vi "Drive Controller.vi"(8 "error in":errorcluster) -> ()   [LabVIEW 2020]
doc: "This VI executes continuously carrying out the current operation and responding to updates or new operation requests. It will often contain the timing or control code that is difficult to place directly in TeleOp. This VI generally opens all sensors and motors and isolates the rest of the robot code from knowing implementation details of how the operations are carried out."
uses:
  <vilib>/Rock Robotics/WPI/Framework/Completion Status.ctl
  Drive Setpoints.ctl
  Drive Operations.ctl
  <vilib>/Rock Robotics/WPI/SafetyOutput/WPI_SafetyOutputConfigMenu.ctl
  <vilib>/Rock Robotics/WPI/RobotDrive/WPI_RobotDriveOpen2MotorWithExistingMotors.vi
  <vilib>/Rock Robotics/Network Tables/NT Write Numeric Array.vi
  <vilib>/Rock Robotics/WPI/ThirdParty/REV Robotics/REVLib/Typedef/Spark MAX Motor Type.ctl
  <vilib>/Rock Robotics/WPI/ThirdParty/REV Robotics/REVLib/Typedef/Spark MAX Idle Mode.ctl
panel:
  in  "Interactive Values":T1
  in  "Buttons":cluster{"Execute Cmd":bool, "Abort Cmd":bool}
  out "Command Timing":cluster{"Start Time (ms)":u32, "Iterations":i32}
  out "Status":T3
  out "Setpoints":T4(graph)
  out "Current\nCmd":string
  # "Tip: The graph shows the motor setpoints. It may also be helpful to observe inputs and sensor values.\nYou may also want to display tuning or debugging controls."
  # "Interactive Command: You may fill in the settings for a command\nand schedule it with the Execute button. You can observe and abort\nany command while fine tuning the code for the controller."
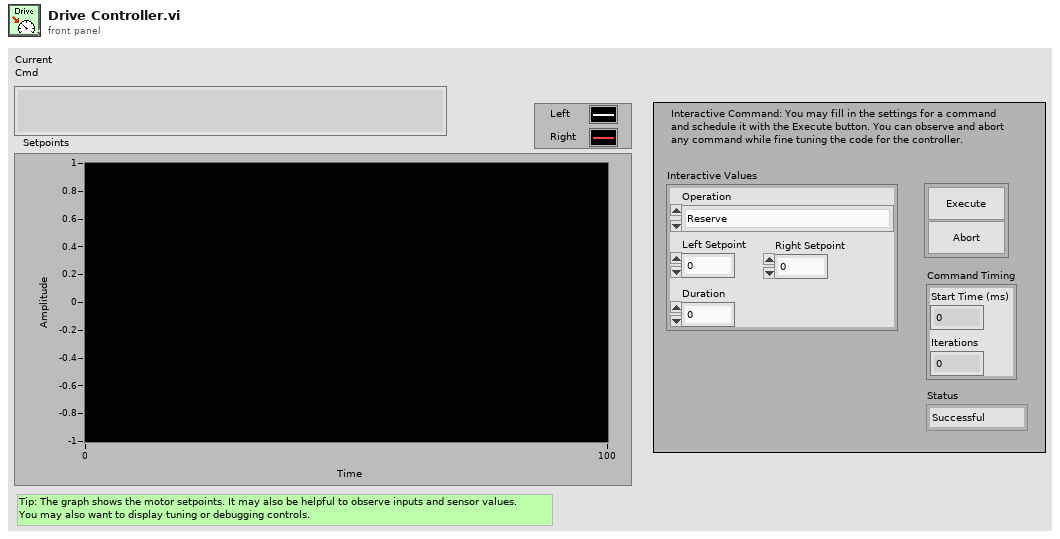
[diagram p1: front panel]
types:
  T1 = typedef "Drive Setpoints.ctl" = cluster{"Operation":T2, "Left Setpoint":dbl, "Right Setpoint":dbl, "Duration":dbl}
  T2 = typedef "Drive Operations.ctl" = enum16{"Reserve", "Read Current", "Immediate", "Drive for Time", "Drive for Distance"}
  T3 = typedef "Completion Status.ctl" = enum16{"Successful", "Aborted", "Incomplete"}
  T4 = cluster{"Left Setpoint":dbl, "Right Setpoint":dbl}
  T5 = typedef "WPI_SafetyOutputConfigMenu.ctl" = enum16{"Enable", "Disable"}
  T6 = typedef "WPI_MotorControlDeviceRef.ctl" = cluster{"DeviceStatus":errorcluster, "Type":T7, "PWM":cluster{"PWM Channel":T8, "DeadBand":T9}, "CAN":cluster{"Device Number":u8, "SetOutput VI Ref":variant, "GetOutput VI Ref":variant, "Enable VI Ref":variant, "Disable VI Ref":variant, "Data":variant}, "Invert":bool, "DIO PWM":cluster{"PWM \"Enable\" Channel":T8, "DIOChannel":T10, "PWM Rate":dbl}}
  T7 = typedef "WPI_MotorControlType.ctl" = enum16{"PWM", "CAN", "DIO PWM"}
  T8 = typedef "FPGA_DIOPWMChannel.ctl" = enum8{"PWM 0", "PWM 1", "PWM 2", "PWM 3", "PWM 4", "PWM 5", "PWM 6", "PWM 7", "PWM 8", "PWM 9", "PWM MXP 0", "PWM MXP 1", "PWM MXP 2", "PWM MXP 3", "PWM MXP 4", "PWM MXP 5", "PWM MXP 6", "PWM MXP 7", "PWM MXP 8", "PWM MXP 9", "Invalid"}
  T9 = typedef "WPI_PWMDeadband.ctl" = cluster{"Name":string, "maxPositivePwm":i32, "minPositivePwm":i32, "centerPwm":i32, "maxNegativePwm":i32, "minNegativePwm":i32, "angularRange":u16}
  T10 = typedef "FPGA_DIOChannel.ctl" = enum8{"DIO 0", "DIO 1", "DIO 2", "DIO 3", "DIO 4", "DIO 5", "DIO 6", "DIO 7", "DIO 8", "DIO 9", "DIO MXP 0", "DIO MXP 1", "DIO MXP 2", "DIO MXP 3", "DIO MXP 4", "DIO MXP 5", "DIO MXP 6", "DIO MXP 7", "DIO MXP 8", "DIO MXP 9", "DIO MXP 10", "DIO MXP 11", "DIO MXP 12", "DIO MXP 13", "DIO MXP 14", "DIO MXP 15", "SPI Port CS1", "SPI Port CS2", "SPI Port CS3", "SPI Port MISO", "SPI Port MOSI", "Invalid"}
  T11 = typedef "Spark MAX Idle Mode.ctl" = enum16{"Coast", "Brake"}
  T12 = typedef "Spark MAX Motor Type.ctl" = enum16{"Brushed", "Brushless"}
  T13 = typedef "WPI_RobotDriveDevRef.ctl" = cluster{"DevStatus":errorcluster, "Motors[]":T6[], "Square Inputs":bool, "Max Output":dbl}
  T14 = typedef "Command Status Info.ctl" = cluster{"Name":string, "Status":T3, "notifier out":T15}
  T15 = typedef "Completion Notifier.ctl" = refnum<notifier>
  T16 = cluster{"SubSystem Data":T1, cluster{"Start Time (ms)":u32, "Iterations":i32}, cluster{"Command Info":T14, "Description":string, "Default Command":T1, "queue out":refnum<queue>, "Subsystem Name":string}}
  T17 = cluster{"SubSystem Data":T1, cluster{"Start Time (ms)":u32, "Iterations":i32}, "Default Command Arguments":cluster{"Command Info":T14, "Description":string, "Default Command":T1, "queue out":refnum<queue>, "Subsystem Name":string}}
  T18 = cluster{"Don't move motors while reserved":dbl, "Don't move motors while reserved":dbl}
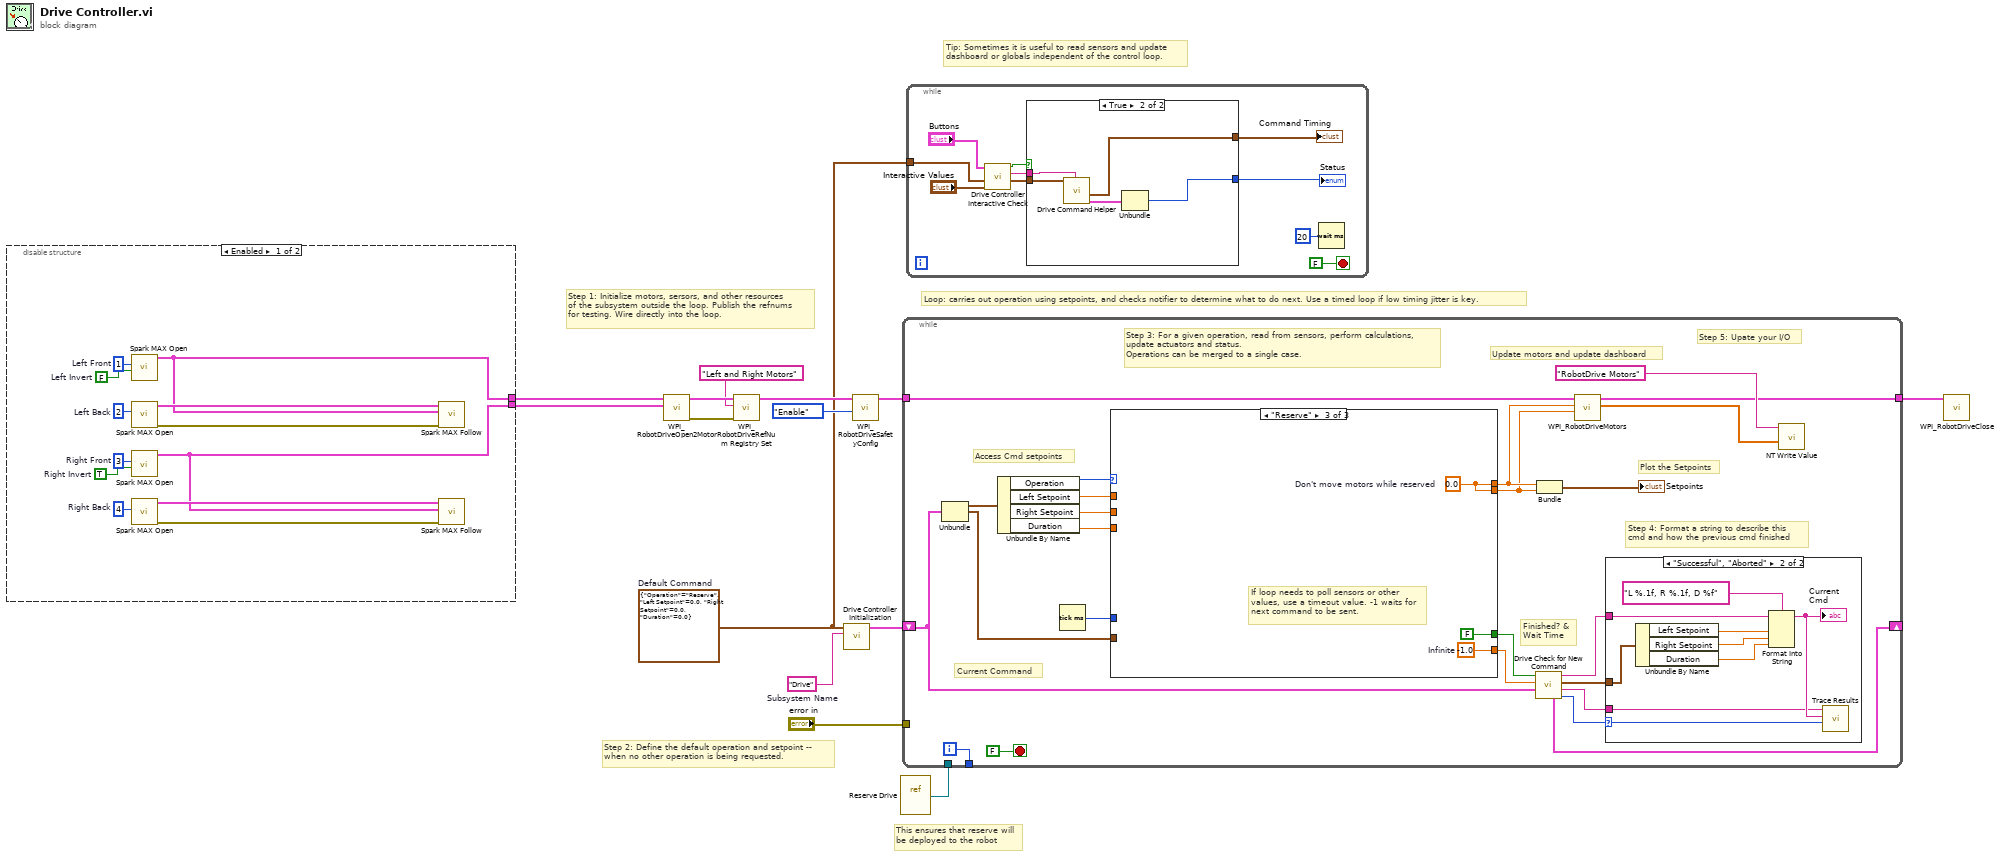
[diagram p0: block diagram]
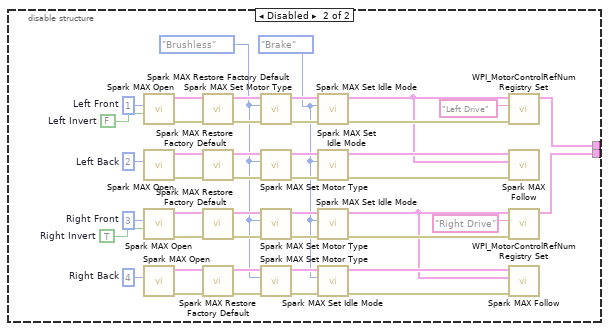
[diagram p2: hidden frame]
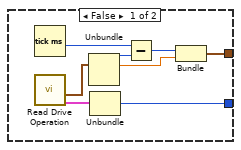
[diagram p3: hidden frame]
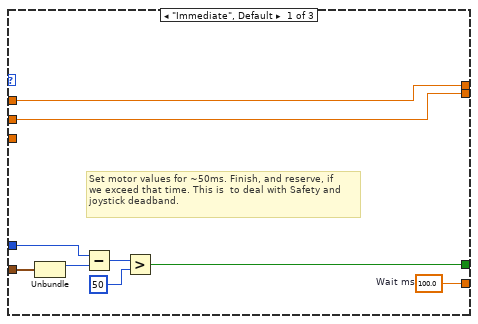
[diagram p5: hidden frame]
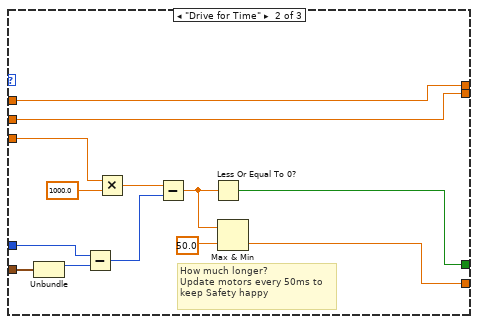
[diagram p6: hidden frame]
diagram:
  w4 = T1 {"Operation"=enum."Reserve", "Left Setpoint"=0.0, "Right Setpoint"=0.0, "Duration"=0.0}  # Default Command
  w14 = "Drive"  # Subsystem Name
  # "This ensures that reserve will\nbe deployed to the robot"
  # "Tip: Sometimes it is useful to read sensors and update\ndashboard or globals independent of the control loop."
  # "Step 2: Define the default operation and setpoint --\nwhen no other operation is being requested."
  # "Step 1: Initialize motors, sersors, and other resources\nof the subsystem outside the loop. Publish the refnums\nfor testing. Wire directly into the loop."
  # "Loop: carries out operation using setpoints, and checks notifier to determine what to do next. Use a timed loop if low timing jitter is key."
  n1 = disable-structure shown="Enabled" {
    disable-tunnel: [w15 w30] -> w3
    disable-tunnel: [w17 w29] -> w2
    frame Enabled {
      w19 = u8 4  # Right Back
      w20 = u8 3  # Right Front
      w21 = u8 2  # Left Back
      w22 = u8 1  # Left Front
      w23 = TRUE  # Right Invert
      w24 = FALSE  # Left Invert
      n2 = call <vilib>:"Spark MAX Open.vi"("Invert"=w24, "Device Number"=w22) -> ("MotorControlDeviceRef"=w15:T6)  [unwired: 8 in, 1 out]
      n3 = call <vilib>:"Spark MAX Open.vi"("Device Number"=w21) -> ("error out"=w26:errorcluster, "MotorControlDeviceRef"=w16:T6)  [unwired: 9 in]
      n4 = call <vilib>:"Spark MAX Open.vi"("Invert"=w23, "Device Number"=w20) -> ("MotorControlDeviceRef"=w17:T6)  [unwired: 8 in, 1 out]
      n5 = call <vilib>:"Spark MAX Open.vi"("Device Number"=w19) -> ("error out"=w25:errorcluster, "MotorControlDeviceRef"=w18:T6)  [unwired: 9 in]
      n6 = call <vilib>:"Spark MAX Follow.vi"("error in (no error)"=w26, "Master Controller"=w15, "MotorControlDeviceRef"=w16) -> ()  [unwired: 7 in, 2 out]
      n7 = call <vilib>:"Spark MAX Follow.vi"("error in (no error)"=w25, "Master Controller"=w17, "MotorControlDeviceRef"=w18) -> ()  [unwired: 7 in, 2 out]
    }
    frame Disabled {
      w27 = Spark_MAX_Idle_Mode."Brake" ("Idle Mode")
      w28 = Spark_MAX_Motor_Type."Brushless" ("Motor Type")
      w37 = u8 4  # Right Back
      w38 = u8 3  # Right Front
      w39 = u8 2  # Left Back
      w40 = u8 1  # Left Front
      w41 = TRUE  # Right Invert
      w42 = FALSE  # Left Invert
      n8 = call <vilib>:"Spark MAX Open.vi"("Invert"=w42, "Device Number"=w40) -> ("error out"=w70:errorcluster, "MotorControlDeviceRef"=w69:T6)  [unwired: 8 in]
      n9 = call <vilib>:"Spark MAX Open.vi"("Device Number"=w39) -> ("error out"=w59:errorcluster, "MotorControlDeviceRef"=w60:T6)  [unwired: 9 in]
      n10 = call <vilib>:"Spark MAX Open.vi"("Invert"=w41, "Device Number"=w38) -> ("error out"=w53:errorcluster, "MotorControlDeviceRef"=w54:T6)  [unwired: 8 in]
      n11 = call <vilib>:"Spark MAX Open.vi"("Device Number"=w37) -> ("error out"=w48:errorcluster, "MotorControlDeviceRef"=w47:T6)  [unwired: 9 in]
      n12 = call <vilib>:"Spark MAX Restore Factory Default.vi"("error in"=w70, "MotorControlDeviceRef"=w69) -> ("error out"=w68:errorcluster, "MotorControlDeviceRef"=w67:T6)  [unwired: 8 in]
      n13 = call <vilib>:"Spark MAX Restore Factory Default.vi"("error in"=w59, "MotorControlDeviceRef"=w60) -> ("error out"=w61:errorcluster, "MotorControlDeviceRef"=w62:T6)  [unwired: 8 in]
      n14 = call <vilib>:"Spark MAX Restore Factory Default.vi"("error in"=w53, "MotorControlDeviceRef"=w54) -> ("error out"=w55:errorcluster, "MotorControlDeviceRef"=w56:T6)  [unwired: 8 in]
      n15 = call <vilib>:"Spark MAX Restore Factory Default.vi"("error in"=w48, "MotorControlDeviceRef"=w47) -> ("error out"=w46:errorcluster, "MotorControlDeviceRef"=w45:T6)  [unwired: 8 in]
      n16 = call <vilib>:"Spark MAX Set Motor Type.vi"("error in (no error)"=w68, "Motor Type"=w28, "MotorControlDevRef"=w67) -> ("error out"=w66:errorcluster, "MotorControlDeviceRef"=w65:T6)  [unwired: 7 in]
      n17 = call <vilib>:"Spark MAX Set Motor Type.vi"("error in (no error)"=w61, "Motor Type"=w28, "MotorControlDevRef"=w62) -> ("error out"=w63:errorcluster, "MotorControlDeviceRef"=w64:T6)  [unwired: 7 in]
      n18 = call <vilib>:"Spark MAX Set Motor Type.vi"("error in (no error)"=w55, "Motor Type"=w28, "MotorControlDevRef"=w56) -> ("error out"=w57:errorcluster, "MotorControlDeviceRef"=w58:T6)  [unwired: 7 in]
      n19 = call <vilib>:"Spark MAX Set Motor Type.vi"("error in (no error)"=w46, "Motor Type"=w28, "MotorControlDevRef"=w45) -> ("error out"=w44:errorcluster, "MotorControlDeviceRef"=w43:T6)  [unwired: 7 in]
      n20 = call <vilib>:"Spark MAX Set Idle Mode.vi"("error in (no error)"=w66, "Idle Mode"=w27, "MotorControlDeviceRef in"=w65) -> ("error out"=w36:errorcluster, "MotorControlDeviceRef out"=w34:T6)  [unwired: 7 in]
      n21 = call <vilib>:"Spark MAX Set Idle Mode.vi"("error in (no error)"=w63, "Idle Mode"=w27, "MotorControlDeviceRef in"=w64) -> ("error out"=w52:errorcluster, "MotorControlDeviceRef out"=w51:T6)  [unwired: 7 in]
      n22 = call <vilib>:"Spark MAX Set Idle Mode.vi"("error in (no error)"=w57, "Idle Mode"=w27, "MotorControlDeviceRef in"=w58) -> ("error out"=w35:errorcluster, "MotorControlDeviceRef out"=w33:T6)  [unwired: 7 in]
      n23 = call <vilib>:"Spark MAX Set Idle Mode.vi"("error in (no error)"=w44, "Idle Mode"=w27, "MotorControlDeviceRef in"=w43) -> ("error out"=w49:errorcluster, "MotorControlDeviceRef out"=w50:T6)  [unwired: 7 in]
      n24 = call <vilib>:"WPI_MotorControlRefNum Registry Set.vi"("error in (no error)"=w36, "refnum name"="Left Drive", "MotorControlDevRef"=w34) -> ("MotorControlDevRef"=w30:T6)  [unwired: 7 in, 1 out]
      n25 = call <vilib>:"Spark MAX Follow.vi"("error in (no error)"=w52, "Master Controller"=w34, "MotorControlDeviceRef"=w51) -> ()  [unwired: 7 in, 2 out]
      n26 = call <vilib>:"WPI_MotorControlRefNum Registry Set.vi"("error in (no error)"=w35, "refnum name"="Right Drive", "MotorControlDevRef"=w33) -> ("MotorControlDevRef"=w29:T6)  [unwired: 7 in, 1 out]
      n27 = call <vilib>:"Spark MAX Follow.vi"("error in (no error)"=w49, "Master Controller"=w33, "MotorControlDeviceRef"=w50) -> ()  [unwired: 7 in, 2 out]
    }
  }
  n28 = call-poly <vilib>:"WPI_RobotDriveOpen2Motor.vi"("Right Motor Dev Ref"=w2, "Left Motor Dev Ref"=w3) -> ("error out"=w11:errorcluster, "RobotDriveDevRef"=w13:T13)  [unwired: 3 in, 5 out]
  n29 = call <vilib>:"WPI_RobotDriveRefNum Registry Set.vi"("error in (no error)"=w11, "refnum name"="Left and Right Motors", "RobotDriveDevRef"=w13) -> ("RobotDriveDevRef"=w10:T13)  [unwired: 1 in, 7 out]
  n30 = call "Drive Controller Initialization.vi"("Subsystem Name"=w14, "Default Command"=w4) -> ("Current Command"=w6:T16)  [unwired: 9 in]
  n31 = call <vilib>:"WPI_RobotDriveSafetyConfig.vi"("mode"=WPI_SafetyOutputConfigMenu."Enable", "RobotDriveDevRef"=w10) -> ("RobotDriveDevRef"=w8:T13)  [unwired: 8 in, 1 out]
  n32 = vi-ref "Reserve Drive.vi"() -> (w5:refnum<vi>)
  n33 = while {
    shift-right: [w81] -> _
    shift-left: w6 -> [w74]
    tunnel: [w93] -> _
    tunnel: w8 -> [w89]
    tunnel: "error in" -> [_]
    tunnel: w5 -> [_]
    tunnel: [w71] -> w1
    i -> [w93]
    stop <- FALSE stop-if-true
    # "Step 5: Upate your I/O"
    # "Step 4: Format a string to describe this\ncmd and how the previous cmd finished"
    # "Current Command"
    # "Update motors and update dashboard"
    # "Plot the Setpoints"
    # "Access Cmd setpoints"
    # "Finished? &\nWait Time"
    # "Step 3: For a given operation, read from sensors, perform calculations,\nupdate actuators and status.\nOperations can be merged to a single case."
    n34 = Unbundle(w74) -> ("SubSystem Data"=w88:T1, w75:cluster{"Start Time (ms)":u32, "Iterations":i32})  [unwired: 1 out]
    n35 = Unbundle By Name(w88) -> ("Operation"=w87:T2, "Left Setpoint"=w86:dbl, "Right Setpoint"=w85:dbl, "Duration"=w84:dbl)
    n36 = Tick Count (ms)() -> (millisecond timer value=w83:u32)
    n37 = case shown="\"Reserve\"" w87 {
      tunnel: [w112 w113 w128] -> w80
      tunnel: [w105 w120 FALSE ("ignore previous (F)")] -> w79
      tunnel: w75 -> [w104 w122 _]
      tunnel: [w111 w119 w126] -> w91
      tunnel: [w110 w118 w126] -> w90
      tunnel: w86 -> [w111 w119 _]
      tunnel: w85 -> [w110 w118 _]
      tunnel: w84 -> [_ w117 _]
      tunnel: w83 -> [w106 w116 _]
      frame "Immediate", Default {
        w112 = 100.0  # Wait ms
        # "Set motor values for ~50ms. Finish, and reserve, if\nwe exceed that time. This is  to deal with Safety and\njoystick deadband."
        n38 = Unbundle(w104) -> ("Start Time (ms)"=w107:u32)  [unwired: 1 out]
        n39 = Subtract(x=w106, y=w107) -> (x-y=w108:u32)
        n40 = Greater?(x=w108, y=u8 50 ("Left Motor")) -> (0:w105:bool)
      }
      frame "Drive for Time" {
        # "How much longer?\nUpdate motors every 50ms to\nkeep Safety happy"
        n41 = Unbundle(w122) -> ("Start Time (ms)"=w121:u32)  [unwired: 1 out]
        n42 = Subtract(x=w116, y=w121) -> (x-y=w125:u32)
        n43 = Multiply(x=w117, y=1000.0) -> (x*y=w124:dbl)
        n44 = Subtract(x=w124, y=w125) -> (x-y=w115:dbl)
        n45 = Less Or Equal To 0?(x=w115) -> (x <= 0?=w120:bool)
        n46 = Max & Min(x=w115, y=50.0) -> (min(x,y)=w113:dbl)  [unwired: 1 out]
      }
      frame "Reserve" {
        w126 = 0.0  # Don't move motors while reserved
        w128 = -1.0  # Infinite
        # "If loop needs to poll sensors or other\nvalues, use a timeout value. -1 waits for\nnext command to be sent."
      }
    }
    n47 = call "Drive Check for New Command.vi"("input cluster"=w74, "Wait time (ms)"=w80, "Finished?"=w79) -> ("Completion"=w82:T3, "Subsystem Name"=w76:string, "Current Command"=w77:T1, "Initial Trace String"=w78:string, "Next Command"=w81:T17)  [unwired: 4 in]
    n48 = Bundle("Don't move motors while reserved"=w91, "Don't move motors while reserved"=w90) -> (→"Setpoints":T18)  [unwired: 1 in]
    n49 = call <vilib>:"WPI_RobotDriveMotors.vi"("RightSpeed"=w90, "LeftSpeed"=w91, "RobotDriveDevRef"=w89) -> ("Motor Values"=w72:dbl[], "RobotDriveDevRef"=w71:T13)  [unwired: 1 in, 6 out]
    n50 = case shown="\"Successful\", \"Aborted\"" w82 {
      selector: w82 -> [_ w103]
      tunnel: w78 -> [_ w98]
      tunnel: w77 -> [_ w99]
      tunnel: w76 -> [_ w95]
      frame "Incomplete", Default {
        # "Continuing current command"
      }
      frame "Successful", "Aborted" {
        # "Report and setup for next command"
        n51 = Unbundle By Name(w99) -> ("Left Setpoint"=w101:dbl, "Right Setpoint"=w102:dbl, "Duration"=w96:dbl)
        n52 = Format Into String(format string="L %.1f, R %.1f, D %f", initial string=w98, w101, w102, w96) -> (resulting string=w97:string)  [unwired: 1 in, 1 out]
        "Current\nCmd" <- w97
        n53 = call <vilib>:"Trace Results.vi"("Status of previous command"=w103, "Description"=w97, "Subsystem"=w95) -> ()  [unwired: 9 in]
      }
    }
    n54 = call-poly <vilib>:"NT Write Value.vi"("Numeric Array"=w72, "Name"="RobotDrive Motors") -> ()  [unwired: 9 in, 1 out]
  }
  n55 = while {
    tunnel: w4 -> [w130]
    stop <- FALSE stop-if-true
    n56 = call "Drive Controller Interactive Check.vi"("Interactive Command In"="Interactive Values", "Default Command"=w130, "Buttons"="Buttons") -> ("Interactive Command Out"=w132:T1, "Trace String"=w133:string, "Schedule"=w134:bool)  [unwired: 6 in]
    n57 = case shown="True" w134 {
      tunnel: [w143 w151] -> w135
      tunnel: [w142 w147] -> w136
      tunnel: w133 -> [_ w149]
      tunnel: w132 -> [_ w148]
      frame False {
        n58 = Tick Count (ms)() -> (millisecond timer value=w146:u32)
        n59 = call "Read Drive Operation.vi"() -> ("Command Info"=w140:T14, "SubSystem Data"=w139:T1)  [unwired: 9 in, 1 out]
        n60 = Unbundle(w139) -> ("Operation"=w144:T2, "Left Setpoint"=w141:dbl)  [unwired: 2 out]
        n61 = Unbundle(w140) -> ("Status"=w143:T3)  [unwired: 2 out]
        n62 = Subtract(x=w146, y=w144) -> (x-y=w145:u32)
        n63 = Bundle(w145, "Left Setpoint"=w141) -> (w142:cluster{u32, "Left Setpoint":dbl})  [unwired: 1 in]
      }
      frame True {
        n64 = call "Drive Command Helper.vi"("Description"=w149, "SubSystem Data"=w148) -> ("Command Info Out"=w150:T14, "Command Timing"=w147:cluster{"Start Time (ms)":u32, "Iterations":i32})  [unwired: 7 in, 1 out]
        n65 = Unbundle(w150) -> ("Status"=w151:T3)  [unwired: 2 out]
      }
    }
    "Status" <- w135
    "Command Timing" <- w136
    n66 = Wait (ms)(milliseconds to wait=u32 20) -> ()  [unwired: 1 out]
  }
  n67 = call <vilib>:"WPI_RobotDriveClose.vi"("RobotDriveDevRef"=w1) -> ()  [unwired: 10 in, 1 out]
